vi "Duty to Ticks.vi"(9 "Duty":dbl, 10 "Frequency":dbl) -> (2 "Ticks":i32)   [LabVIEW 2019]
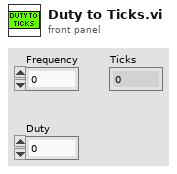
[diagram p1: front panel]
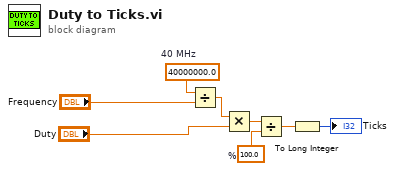
[diagram p0: block diagram]
diagram:
  w6 = 40000000.0  # 40 MHz
  w3 = 100.0  # %
  n1 = Divide(x=w6, y="Frequency") -> (x/y=w1:dbl)
  n2 = Multiply(x=w1, y="Duty") -> (x*y=w2:dbl)
  n3 = Divide(x=w2, y=w3) -> (x/y=w4:dbl)
  n4 = To Long Integer(number=w4) -> (32bit integer=→"Ticks":i32)
